vi "Lockin.DAQ.Read AI.vi"(8 "error in (no error)":errorcluster, 10 "AO []":waveform(dbl)[](array[waveform]), 11 "Lockin.DAQ in":refnum<class "Instrument.DAQ.lvclass">) -> (0 "error out":errorcluster, 1 "AI time (ms)":u32=2, 2 "AI []":waveform(dbl)[](array[waveform]), 3 "Lockin.DAQ out":refnum<class "Instrument.DAQ.lvclass">)   [LabVIEW 2019, in "Instrument.DAQ.lvclass"]
uses:
  Instrument.DAQ.lvclass
  Instrument.DAQ.lvclass/Instrument.DAQ.ctl
  Typedefs/AI Simulation-enum.ctl
  Waveguide Model/Waveguide Model--Cluster.ctl
  <vilib>/DAQmx/read.llb/DAQmx Read (Analog 1D Wfm NChan NSamp).vi
  <vilib>/DAQmx/miscellaneous.llb/DAQmx Fill In Error Info.vi
  <userlib>/_OpenG.lib/array/array.llb/Reorder 1D Array2 (Variant)__ogtk.vi
  <userlib>/_OpenG.lib/array/array.llb/Sort 1D Array (I32)__ogtk.vi
  <resource>/objmgr/daqmx.rc
panel:
  out "P Check":bool[](array[boolean])
  out "time to read samples":u32
  out "time to check for samples":u32
  out "Numeric":i32
  out "AvailSampPerChan 4":u32
  out "AvailSampPerChan 3":u32
  out "AvailSampPerChan 2":u32
  out "AvailSampPerChan 1":u32
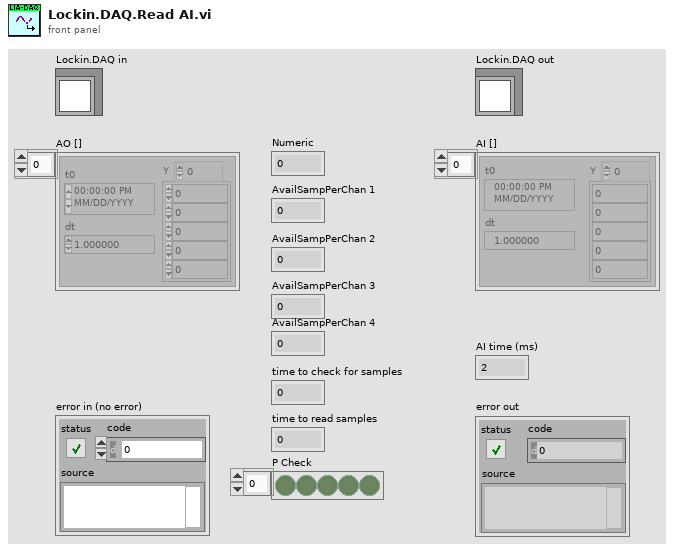
[diagram p1: front panel]
types:
  T1 = typedef "Instrument.DAQ.lvclass/AI Simulation-enum.ctl" = enum16{"AI = HW simulated", "AI = noise*AO", "AI = waveguide"}
  T2 = typedef "Instrument.DAQ.lvclass/Waveguide Model--Cluster.ctl" = cluster{"Vsource Index":i32, "Vsg Index":i32, "V+":i32, "V-":i32}
  T3 = enum16{"static", "dynamic", "dynamic asynchronous"}
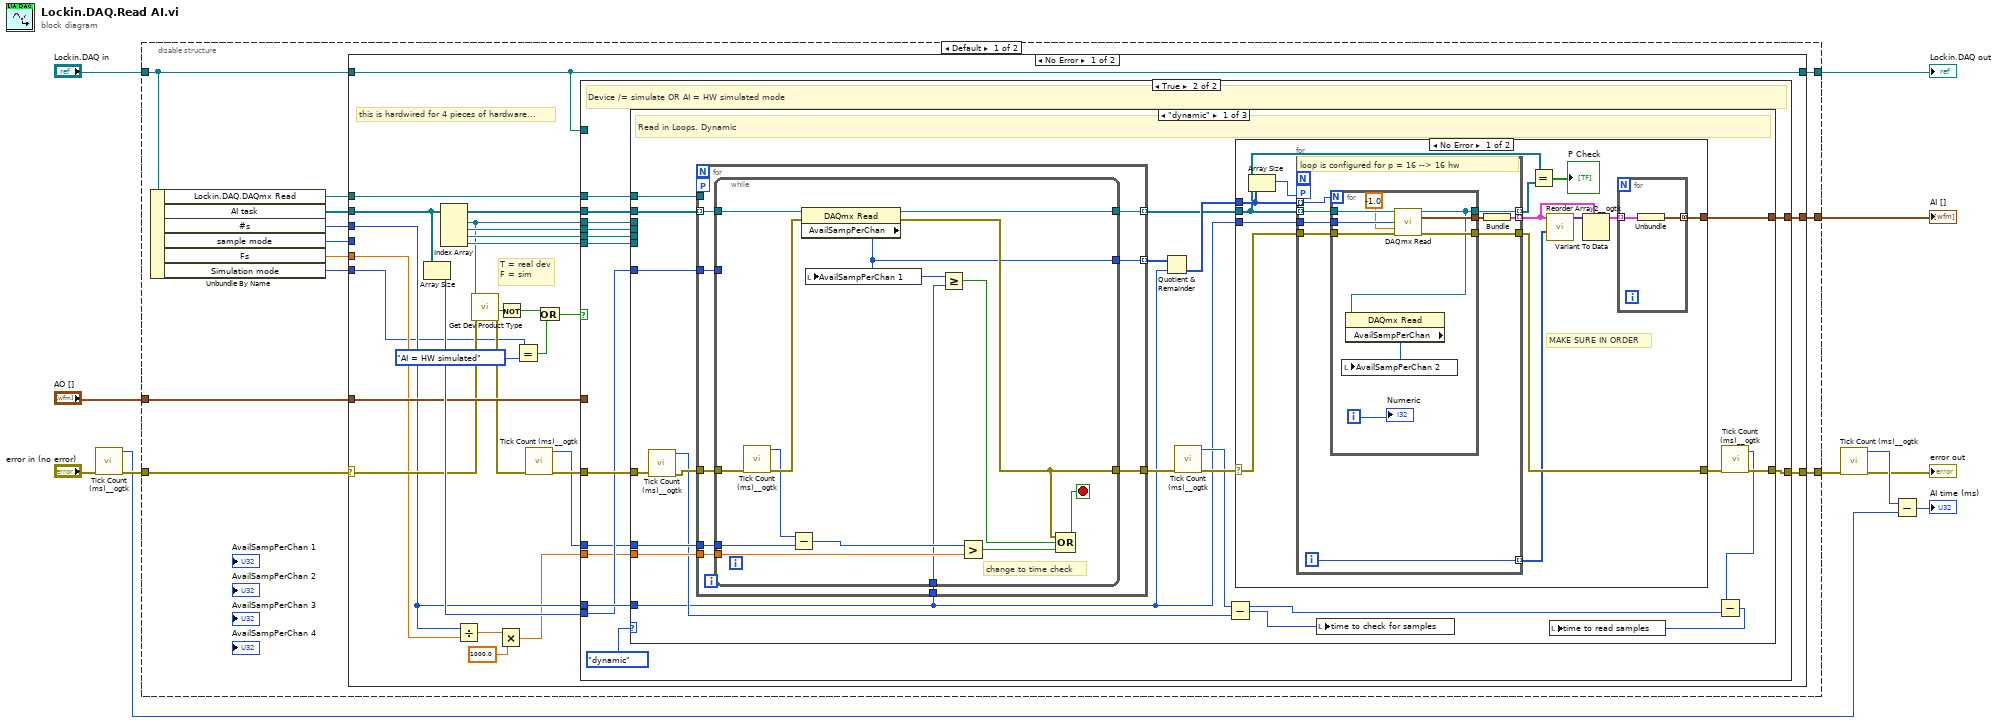
[diagram p0: block diagram]
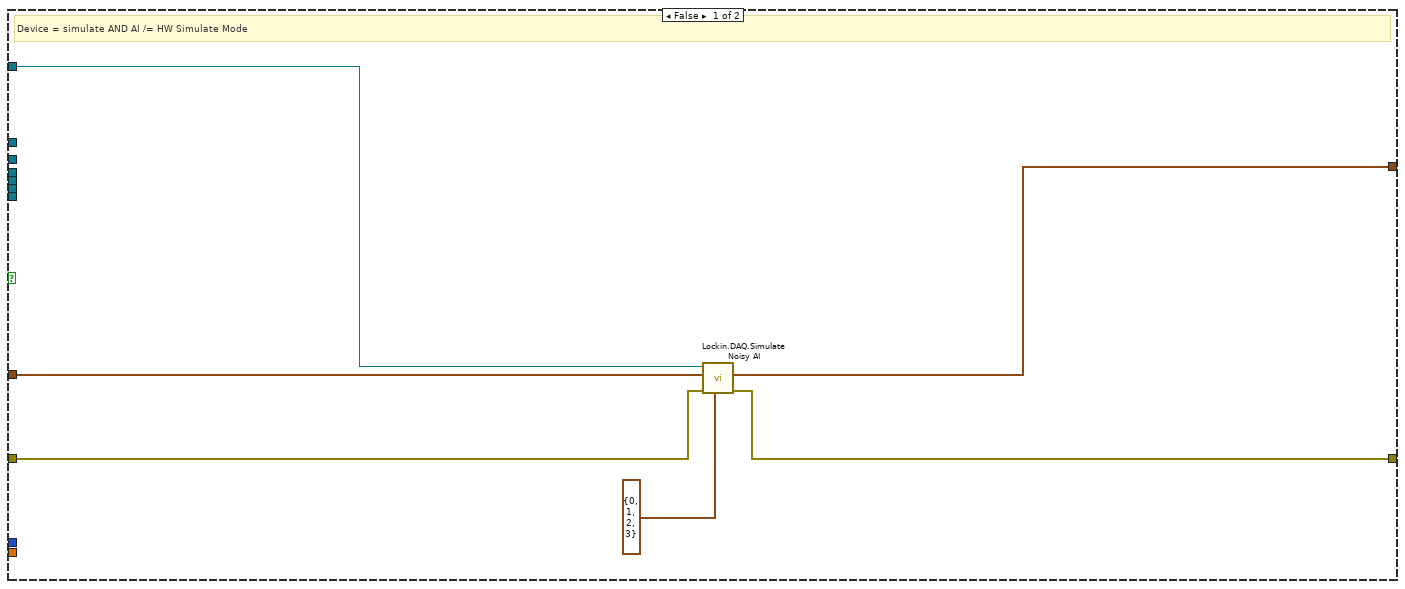
[diagram p2: hidden frame]
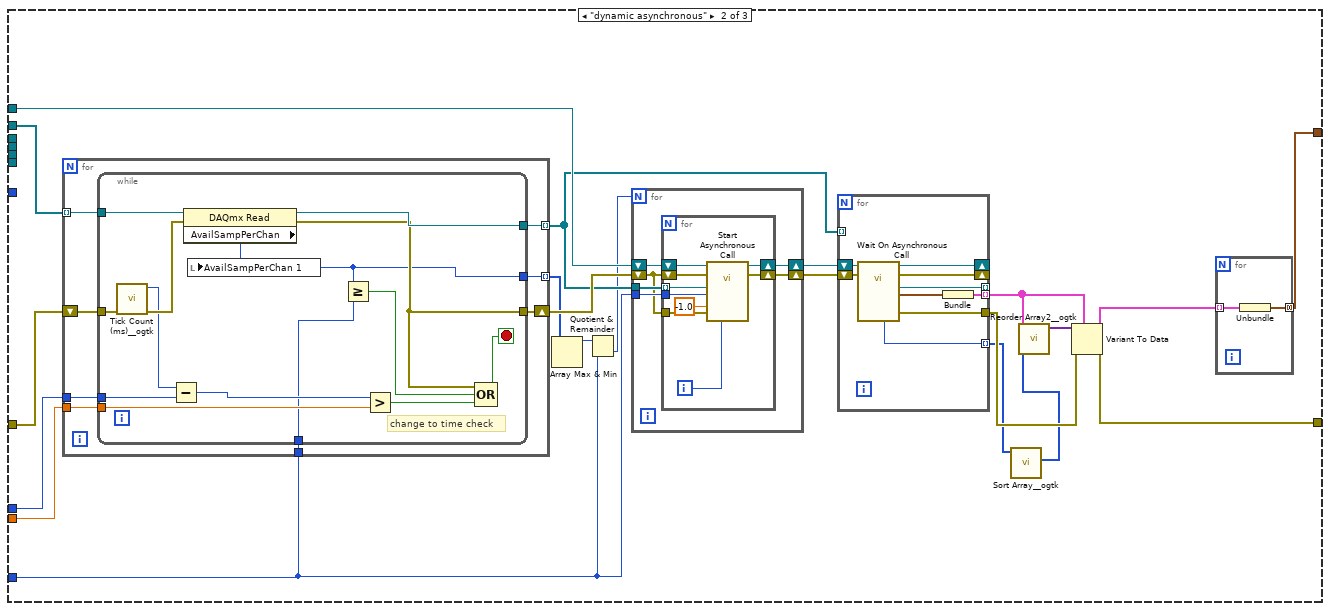
[diagram p4: hidden frame]
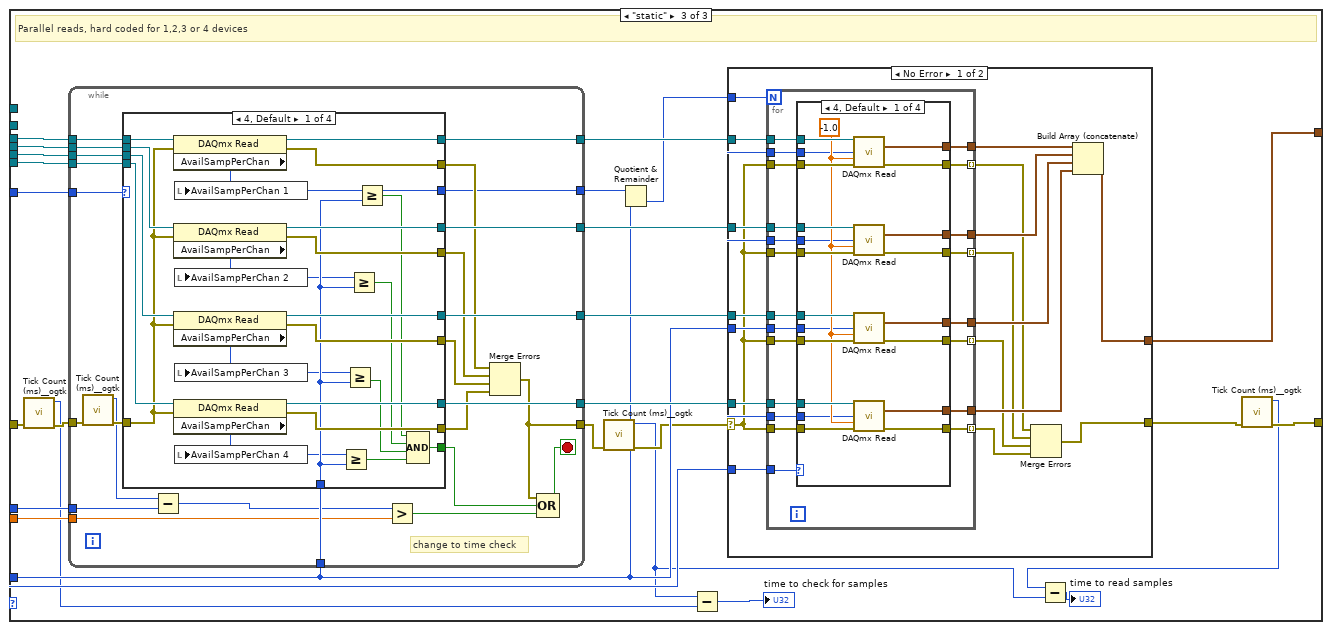
[diagram p5: hidden frame]
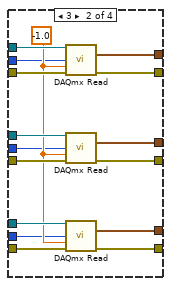
[diagram p6: hidden frame]
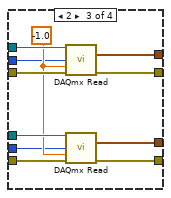
[diagram p7: hidden frame]
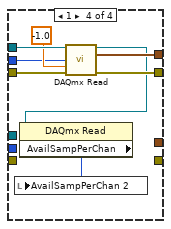
[diagram p8: hidden frame]
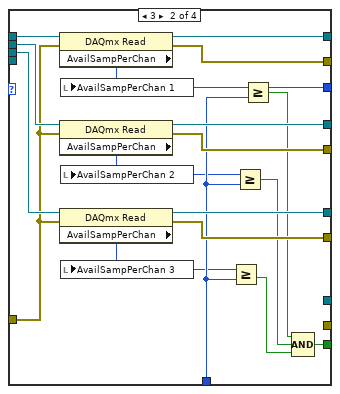
[diagram p10: hidden frame]
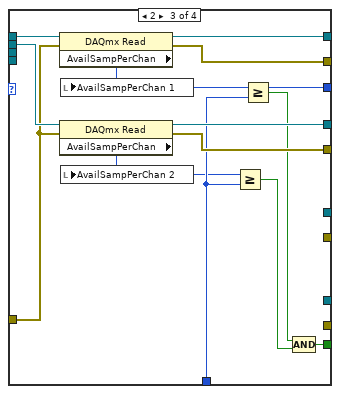
[diagram p11: hidden frame]
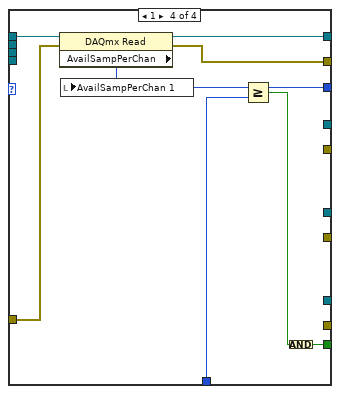
[diagram p12: hidden frame]
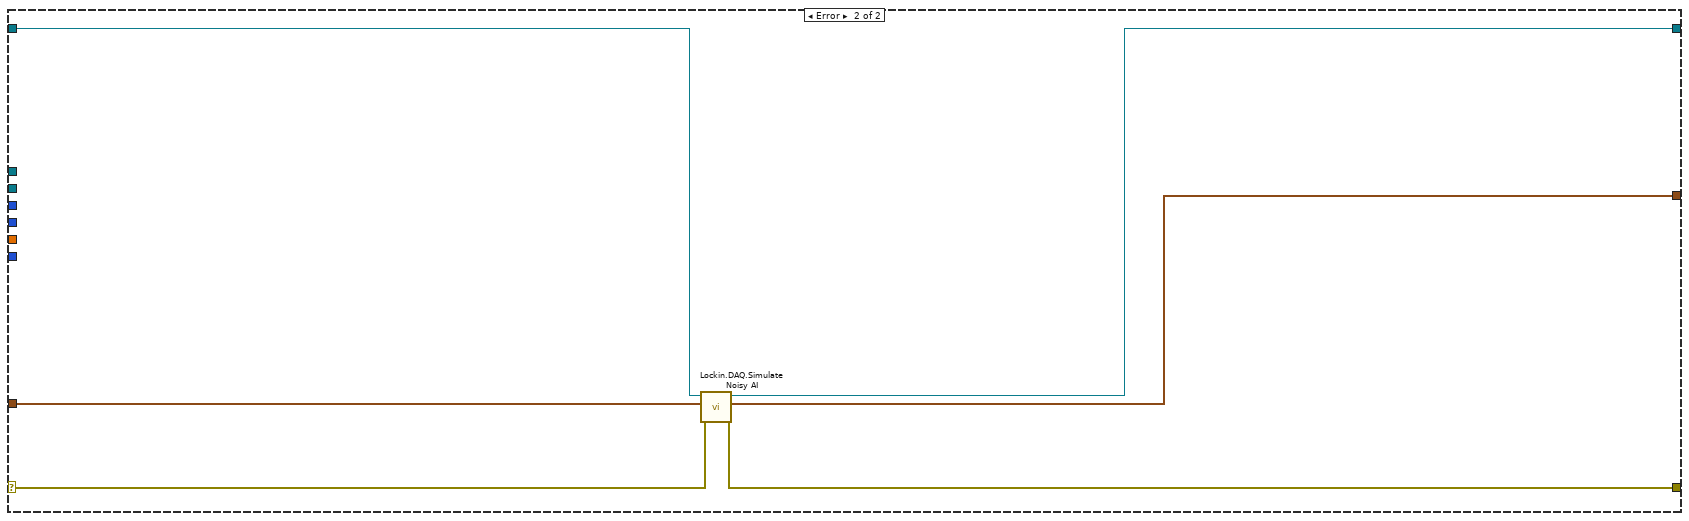
[diagram p13: hidden frame]
diagram:
  n1 = call <userlib>:"Tick Count (ms)__ogtk.vi"("error in (no error)"="error in (no error)") -> ("error out"=w8:errorcluster, "millisecond timer value"=w3:u32)  [unwired: 9 in]
  n2 = disable-structure shown="Default" {
    disable-tunnel: [w23 w432] -> w1
    disable-tunnel: [w20 w433] -> w7
    disable-tunnel: "Lockin.DAQ in" -> [w18 _]
    disable-tunnel: "AO []" -> [w19 w432]
    disable-tunnel: w8 -> [w14 w433]
    disable-tunnel: [w17 _] -> w10
    frame condition #0 (active) {
      n3 = Unbundle By Name(w18) -> ("Lockin.DAQ.DAQmx Read"=w13:refnum<vi>, "AI task"=w16:refnum<k21>[], "#s"=w22:i32, "sample mode"=w21:i32, "Fs"=w15:dbl, "Simulation mode"=w12:T1)
      n4 = case shown="No Error" w14 {
        selector: w14 -> [w40 w427]
        tunnel: [w49 w430] -> w23
        tunnel: w22 -> [w39 _]
        tunnel: w21 -> [_ _]
        tunnel: [w41 w429] -> w20
        tunnel: w19 -> [w44 w428]
        tunnel: w16 -> [w31 _]
        tunnel: w18 -> [w43 w426]
        tunnel: [w43 w431] -> w17
        tunnel: w15 -> [w38 _]
        tunnel: w13 -> [w30 _]
        tunnel: w12 -> [w24 _]
        frame No Error {
          # "T = real dev\nF = sim"
          # "this is hardwired for 4 pieces of hardware..."
          n5 = Array Size(array=w31) -> (size(s)=w45:i32)
          n6 = Index Array(array=w31) -> (element #1=w42:refnum<k21>, element #2=w46:refnum<k21>, element #3=w47:refnum<k21>, element #4=w48:refnum<k21>)  [unwired: 4 in]
          n7 = Divide(x=w39, y=w38) -> (x/y=w37:dbl)
          n8 = call "Get Dev Product Type.vi"("error in (no error)"=w40, "Refnum in"=w42) -> ("error out"=w34:errorcluster, "DevIsSimulated"=w27:bool)  [unwired: 6 in, 2 out]
          n9 = Multiply(x=w37, y=1000.0) -> (x*y=w33:dbl)
          n10 = Not(x=w27) -> (.not. x?=w25:bool)
          n11 = Equal?(x=w24, y=AI_Simulation-enum."AI = HW simulated") -> (x = y?=w28:bool)
          n12 = call <userlib>:"Tick Count (ms)__ogtk.vi"("error in (no error)"=w34) -> ("error out"=w35:errorcluster, "millisecond timer value"=w32:u32)  [unwired: 9 in]
          n13 = Or(x=w25, y=w28) -> (x .or. y?=w26:bool)
          n14 = case shown="True" w26 {
            tunnel: [w53 w69] -> w49
            tunnel: w48 -> [_ w68]
            tunnel: w47 -> [_ w67]
            tunnel: w46 -> [_ w66]
            tunnel: w42 -> [_ w65]
            tunnel: w39 -> [_ w64]
            tunnel: w35 -> [w51 w62]
            tunnel: w45 -> [_ w61]
            tunnel: [w50 w63] -> w41
            tunnel: w44 -> [w55 _]
            tunnel: w43 -> [w54 _]
            tunnel: w33 -> [_ w60]
            tunnel: w32 -> [_ w59]
            tunnel: w31 -> [_ w58]
            tunnel: w30 -> [_ w57]
            frame False {
              # "Device = simulate AND AI /= HW Simulate Mode"
              n15 = call "Lockin.DAQ.Simulate Noisy AI.vi"("Waveguide Cluster"=T2 {"Vsource Index"=0, "Vsg Index"=1, "V+"=2, "V-"=3}, "error in (no error)"=w51, "AO []"=w55, "Lockin.DAQ in"=w54) -> ("error out"=w50:errorcluster, "Noisy AI []"=w53:waveform(dbl)[])  [unwired: 5 in, 1 out]
            }
            frame True {
              # "Device /= simulate OR AI = HW simulated mode"
              n16 = case shown="\"dynamic\"" T3."dynamic" ("Enum") {
                tunnel: [w90 w166 w242] -> w69
                tunnel: w68 -> [_ _ w241]
                tunnel: w67 -> [_ _ w240]
                tunnel: w66 -> [_ _ w239]
                tunnel: w65 -> [_ _ w238]
                tunnel: w64 -> [w70 w157 w233]
                tunnel: [w79 w150 w221] -> w63
                tunnel: w62 -> [w81 w163 w225]
                tunnel: w61 -> [w85 _ w232]
                tunnel: w60 -> [w89 w161 w231]
                tunnel: w59 -> [w86 w162 w228]
                tunnel: w58 -> [w84 w165 _]
                tunnel: w57 -> [w82 w160 _]
                frame "dynamic" {
                  # "Read in Loops. Dynamic"
                  n17 = call <userlib>:"Tick Count (ms)__ogtk.vi"("error in (no error)"=w81) -> ("error out"=w80:errorcluster, "millisecond timer value"=w75:u32)  [unwired: 9 in]
                  n18 = for {
                    tunnel: w70 -> [w99]
                    tunnel: w89 -> [w97]
                    tunnel: w85 -> [w93]
                    tunnel: w84 -> [w92] mode=indexing
                    tunnel: w86 -> [w94]
                    tunnel: [w96] -> w87 mode=indexing
                    tunnel: [w91] -> w83 mode=indexing
                    tunnel: w82 -> [_]
                    workers-P: _ -> [_]
                    tunnel: w80 -> [w98]
                    tunnel: [w95] -> w78
                    n19 = while {
                      tunnel: [w113] -> w91
                      tunnel: w98 -> [w108]
                      tunnel: [w111] -> w95
                      tunnel: w99 -> [w100]
                      tunnel: w93 -> [_]
                      tunnel: w97 -> [w109]
                      tunnel: [w101] -> w96
                      tunnel: w94 -> [w105]
                      tunnel: w92 -> [w102]
                      stop <- w112 stop-if-true
                      # "change to time check"
                      n20 = call <userlib>:"Tick Count (ms)__ogtk.vi"("error in (no error)"=w108) -> ("error out"=w107:errorcluster, "millisecond timer value"=w106:u32)  [unwired: 9 in]
                      n21 = Subtract(x=w106, y=w105) -> (x-y=w104:u32)
                      n22 = property class="DAQmx Read"(reference=w102, error in=w107) -> (reference out=w113:refnum<k21>, error out=w111:errorcluster, "AvailSampPerChan"=w101:u32)
                      n23 = local write "AvailSampPerChan 1"(w101) -> ()
                      n24 = Greater Or Equal?(x=w101, y=w100) -> (x >= y?=w103:bool)
                      n25 = Greater?(x=w104, y=w109) -> (0:w110:bool)
                      n26 = Compound Arithmetic op=OR(w111, w103, w110) -> (w112:bool)
                    }
                  }
                  n27 = Quotient & Remainder(x=w87, y=w70) -> (floor(x/y)=w88:u32[])  [unwired: 1 out]
                  n28 = call <userlib>:"Tick Count (ms)__ogtk.vi"("error in (no error)"=w78) -> ("error out"=w77:errorcluster, "millisecond timer value"=w71:u32)  [unwired: 9 in]
                  n29 = Subtract(x=w71, y=w75) -> (x-y=w73:u32)
                  n30 = case shown="No Error" w77 {
                    selector: w77 -> [w125 w147]
                    tunnel: [w118 _] -> w90
                    tunnel: w70 -> [w126 _]
                    tunnel: [w122 w147] -> w76
                    tunnel: w88 -> [w124 _]
                    tunnel: w83 -> [w115 _]
                    frame No Error {
                      # "MAKE SURE IN ORDER"
                      n31 = Array Size(array=w124) -> (size(s)=w123:i32)
                      n32 = for {
                        N: w123 -> [_]
                        tunnel: w126 -> [w137]
                        tunnel: [w130] -> w117 mode=indexing
                        tunnel: w124 -> [w132] mode=indexing
                        tunnel: w125 -> [w135]
                        tunnel: [w134] -> w122
                        tunnel: w115 -> [w133] mode=indexing
                        workers-P: w123 -> [_]
                        tunnel: [w131] -> w119 mode=indexing
                        tunnel: [w129] -> w116 mode=indexing
                        i -> [w131]
                        # "loop is configured for p = 16 --> 16 hw"
                        n33 = for {
                          N: w132 -> [_]
                          tunnel: w133 -> [w146]
                          tunnel: w135 -> [w145]
                          tunnel: [w144] -> w136
                          tunnel: w137 -> [w143]
                          tunnel: [w142] -> w134
                          tunnel: [w138] -> w129
                          i -> [w141]
                          n34 = call-poly <vilib>:"DAQmx Read.vi"("task/channels in"=w146, "number of samples per channel"=w143, "timeout"=-1.0, "error in"=w145) -> ("task out"=w138:refnum<k21>, "data"=w144:waveform(dbl)[], "error out"=w142:errorcluster)  [unwired: 9 in]
                          n35 = property class="DAQmx Read"(reference=w138) -> ("AvailSampPerChan"=w139:u32)  [unwired: 1 in, 2 out]
                          n36 = local write "AvailSampPerChan 2"(w139) -> ()
                          "Numeric" <- w141
                        }
                        n37 = Bundle("data"=w136) -> (w130:cluster{"data":waveform(dbl)[]})  [unwired: 1 in]
                      }
                      n38 = Equal?(x=w115, y=w116) -> (x = y?=→"P Check":bool[])
                      n39 = call-poly <userlib>:"Reorder Array2__ogtk.vi"("indices"=w119, "array"=w117) -> ("reordered array"=w121:variant[])  [unwired: 9 in]
                      n40 = Variant To Data(type=w117, Variant=w121) -> (data=w120:cluster{"data":waveform(dbl)[]}[])  [unwired: 1 in, 1 out]
                      n41 = for {
                        tunnel: w120 -> [w128] mode=indexing
                        tunnel: [w127] -> w118 mode=concatenating
                        n42 = Unbundle(w128) -> ("data"=w127:waveform(dbl)[])
                      }
                    }
                    frame Error {
                    }
                  }
                  n43 = local write "time to check for samples"(w73) -> ()
                  n44 = call <userlib>:"Tick Count (ms)__ogtk.vi"("error in (no error)"=w76) -> ("error out"=w79:errorcluster, "millisecond timer value"=w74:u32)  [unwired: 9 in]
                  n45 = Subtract(x=w74, y=w71) -> (x-y=w72:u32)
                  n46 = local write "time to read samples"(w72) -> ()
                }
                frame "dynamic asynchronous" {
                  n47 = for {
                    tunnel: w157 -> [w191]
                    tunnel: w161 -> [w189]
                    shift-right: [w187] -> w164
                    shift-left: w163 -> [w190]
                    tunnel: w165 -> [w185] mode=indexing
                    tunnel: w162 -> [w186]
                    tunnel: [w188] -> w159 mode=indexing
                    tunnel: [w184] -> w156 mode=indexing
                    n48 = while {
                      tunnel: [w205] -> w184
                      tunnel: w190 -> [w200]
                      tunnel: [w203] -> w187
                      tunnel: w191 -> [w192]
                      tunnel: w189 -> [w201]
                      tunnel: [w193] -> w188
                      tunnel: w186 -> [w197]
                      tunnel: w185 -> [w194]
                      stop <- w204 stop-if-true
                      # "change to time check"
                      n49 = call <userlib>:"Tick Count (ms)__ogtk.vi"("error in (no error)"=w200) -> ("error out"=w199:errorcluster, "millisecond timer value"=w198:u32)  [unwired: 9 in]
                      n50 = Subtract(x=w198, y=w197) -> (x-y=w196:u32)
                      n51 = property class="DAQmx Read"(reference=w194, error in=w199) -> (reference out=w205:refnum<k21>, error out=w203:errorcluster, "AvailSampPerChan"=w193:u32)
                      n52 = local write "AvailSampPerChan 1"(w193) -> ()
                      n53 = Greater Or Equal?(x=w193, y=w192) -> (x >= y?=w195:bool)
                      n54 = Greater?(x=w196, y=w201) -> (0:w202:bool)
                      n55 = Compound Arithmetic op=OR(w203, w195, w202) -> (w204:bool)
                    }
                  }
                  n56 = Array Max & Min(array=w159) -> (max value=w158:u32)  [unwired: 3 out]
                  n57 = Quotient & Remainder(x=w158, y=w157) -> (floor(x/y)=w155:u32)  [unwired: 1 out]
                  n58 = for {
                    N: w155 -> [_]
                    tunnel: w156 -> [w172]
                    tunnel: w157 -> [w170]
                    shift-right: [w173] -> w167
                    shift-left: w164 -> [w169]
                    shift-right: [w174] -> w168
                    shift-left: w160 -> [w171]
                    n59 = for {
                      shift-right: [w183] -> w173
                      shift-left: w169 -> [w180]
                      shift-right: [w182] -> w174
                      shift-left: w171 -> [w181]
                      tunnel: w169 -> [w179]
                      tunnel: w172 -> [w178] mode=indexing
                      tunnel: w170 -> [w176]
                      i -> [w175]
                      n60 = call-by-ref "Start Asynchronous Call"(reference=w181, error in=w180, "Refnum in"=w178, "number of samples per channel"=w176, "timeout"=-1.0, 11:"error in (no error)"=w179, "ID in"=w175) -> (reference out=w182:refnum<vi>, error out=w183:errorcluster)  [unwired: 7 in, 4 out]
                    }
                  }
                  n61 = for {
                    shift-right: [w211] -> _
                    shift-left: w167 -> [w213]
                    shift-right: [w212] -> _
                    shift-left: w168 -> [w214]
                    tunnel: [w208] -> _ mode=indexing
                    tunnel: [w210] -> w151
                    tunnel: [w207] -> w153 mode=indexing
                    tunnel: [w206] -> w149 mode=indexing
                    tunnel: w156 -> [_] mode=indexing
                    n62 = call-by-ref "Wait On Asynchronous Call"(reference=w214, error in=w213) -> (reference out=w212:refnum<vi>, error out=w211:errorcluster, "Refnum out"=w208:refnum<k21>, "data"=w209:waveform(dbl)[], "ID out"=w206:i32, 15:"error out"=w210:errorcluster)  [unwired: 12 in]
                    n63 = Bundle("data"=w209) -> (w207:cluster{"data":waveform(dbl)[]})  [unwired: 1 in]
                  }
                  n64 = call-poly <userlib>:"Sort Array__ogtk.vi"("Array in"=w149) -> ("Sorted Pointers"=w148:i32[])  [unwired: 9 in, 1 out]
                  n65 = call-poly <userlib>:"Reorder Array2__ogtk.vi"("indices"=w148, "array"=w153) -> ("reordered array"=w154:variant[])  [unwired: 9 in]
                  n66 = Variant To Data(error in=w151, type=w153, Variant=w154) -> (data=w152:cluster{"data":waveform(dbl)[]}[], error out=w150:errorcluster)
                  n67 = for {
                    tunnel: [w216] -> w166 mode=concatenating
                    tunnel: w152 -> [w215] mode=indexing
                    n68 = Unbundle(w215) -> ("data"=w216:waveform(dbl)[])
                  }
                }
                frame "static" {
                  # "Parallel reads, hard coded for 1,2,3 or 4 devices"
                  n69 = call <userlib>:"Tick Count (ms)__ogtk.vi"("error in (no error)"=w225) -> ("error out"=w224:errorcluster, "millisecond timer value"=w223:u32)  [unwired: 9 in]
                  n70 = while {
                    tunnel: w241 -> [w363]
                    tunnel: w240 -> [w362]
                    tunnel: w239 -> [w361]
                    tunnel: w238 -> [w360]
                    tunnel: [w359] -> w237
                    tunnel: [w358] -> w236
                    tunnel: [w357] -> w235
                    tunnel: [w356] -> w234
                    tunnel: w224 -> [w343]
                    tunnel: [w345] -> w227
                    tunnel: w233 -> [w355]
                    tunnel: w232 -> [w354]
                    tunnel: w231 -> [w347]
                    tunnel: [w344] -> w229
                    tunnel: w228 -> [w340]
                    stop <- w353 stop-if-true
                    # "change to time check"
                    n71 = call <userlib>:"Tick Count (ms)__ogtk.vi"("error in (no error)"=w343) -> ("error out"=w342:errorcluster, "millisecond timer value"=w341:u32)  [unwired: 9 in]
                    n72 = case shown="4, Default" w354 {
                      tunnel: w363 -> [w386 _ _ _]
                      tunnel: w362 -> [w385 w404 _ _]
                      tunnel: w361 -> [w384 w403 w417 _]
                      tunnel: w360 -> [w383 w402 w416 w425]
                      tunnel: [w382 w401 w415 w424] -> w359
                      tunnel: [w381 w400 w414 _] -> w358
                      tunnel: [w380 w399 _ _] -> w357
                      tunnel: [w379 _ _ _] -> w356
                      tunnel: [w378 w398 w413 w423] -> w349
                      tunnel: [w377 w397 w412 _] -> w350
                      tunnel: [w376 w396 _ _] -> w351
                      tunnel: [w375 _ _ _] -> w352
                      tunnel: w342 -> [w374 w395 w411 w422]
                      tunnel: w355 -> [w369 w391 w408 w420]
                      tunnel: [w365 w388 w406 w419] -> w346
                      tunnel: [w364 w387 w405 w418] -> w344
                      frame 4, Default {
                        n73 = property class="DAQmx Read"(reference=w383, error in=w374) -> (reference out=w382:refnum<k21>, error out=w378:errorcluster, "AvailSampPerChan"=w364:u32)
                        n74 = property class="DAQmx Read"(reference=w384, error in=w374) -> (reference out=w381:refnum<k21>, error out=w377:errorcluster, "AvailSampPerChan"=w366:u32)
                        n75 = property class="DAQmx Read"(reference=w385, error in=w374) -> (reference out=w380:refnum<k21>, error out=w376:errorcluster, "AvailSampPerChan"=w367:u32)
                        n76 = property class="DAQmx Read"(reference=w386, error in=w374) -> (reference out=w379:refnum<k21>, error out=w375:errorcluster, "AvailSampPerChan"=w368:u32)
                        n77 = local write "AvailSampPerChan 1"(w364) -> ()
                        n78 = local write "AvailSampPerChan 2"(w366) -> ()
                        n79 = local write "AvailSampPerChan 3"(w367) -> ()
                        n80 = local write "AvailSampPerChan 4"(w368) -> ()
                        n81 = Greater Or Equal?(x=w368, y=w369) -> (x >= y?=w373:bool)
                        n82 = Greater Or Equal?(x=w367, y=w369) -> (x >= y?=w372:bool)
                        n83 = Greater Or Equal?(x=w366, y=w369) -> (x >= y?=w371:bool)
                        n84 = Greater Or Equal?(x=w364, y=w369) -> (x >= y?=w370:bool)
                        n85 = Compound Arithmetic op=AND(w370, w371, w372, w373) -> (w365:bool)
                      }
                      frame 3 {
                        n86 = property class="DAQmx Read"(reference=w402, error in=w395) -> (reference out=w401:refnum<k21>, error out=w398:errorcluster, "AvailSampPerChan"=w387:u32)
                        n87 = property class="DAQmx Read"(reference=w403, error in=w395) -> (reference out=w400:refnum<k21>, error out=w397:errorcluster, "AvailSampPerChan"=w389:u32)
                        n88 = property class="DAQmx Read"(reference=w404, error in=w395) -> (reference out=w399:refnum<k21>, error out=w396:errorcluster, "AvailSampPerChan"=w390:u32)
                        n89 = local write "AvailSampPerChan 1"(w387) -> ()
                        n90 = local write "AvailSampPerChan 2"(w389) -> ()
                        n91 = local write "AvailSampPerChan 3"(w390) -> ()
                        n92 = Greater Or Equal?(x=w390, y=w391) -> (x >= y?=w394:bool)
                        n93 = Greater Or Equal?(x=w389, y=w391) -> (x >= y?=w393:bool)
                        n94 = Greater Or Equal?(x=w387, y=w391) -> (x >= y?=w392:bool)
                        n95 = Compound Arithmetic op=AND(w392, w393, w394) -> (w388:bool)
                      }
                      frame 2 {
                        n96 = property class="DAQmx Read"(reference=w416, error in=w411) -> (reference out=w415:refnum<k21>, error out=w413:errorcluster, "AvailSampPerChan"=w405:u32)
                        n97 = property class="DAQmx Read"(reference=w417, error in=w411) -> (reference out=w414:refnum<k21>, error out=w412:errorcluster, "AvailSampPerChan"=w407:u32)
                        n98 = local write "AvailSampPerChan 1"(w405) -> ()
                        n99 = local write "AvailSampPerChan 2"(w407) -> ()
                        n100 = Greater Or Equal?(x=w407, y=w408) -> (x >= y?=w410:bool)
                        n101 = Greater Or Equal?(x=w405, y=w408) -> (x >= y?=w409:bool)
                        n102 = Compound Arithmetic op=AND(w409, w410) -> (w406:bool)
                      }
                      frame 1 {
                        n103 = property class="DAQmx Read"(reference=w425, error in=w422) -> (reference out=w424:refnum<k21>, error out=w423:errorcluster, "AvailSampPerChan"=w418:u32)
                        n104 = local write "AvailSampPerChan 1"(w418) -> ()
                        n105 = Greater Or Equal?(x=w418, y=w420) -> (x >= y?=w421:bool)
                        n106 = Compound Arithmetic op=AND(w421) -> (w419:bool)
                      }
                    }
                    n107 = Subtract(x=w341, y=w340) -> (x-y=w339:u32)
                    n108 = Greater?(x=w339, y=w347) -> (0:w348:bool)
                    n109 = Merge Errors(w349, w350, w351, w352) -> (w345:errorcluster)
                    n110 = Compound Arithmetic op=OR(w345, w346, w348) -> (w353:bool)
                  }
                  n111 = call <userlib>:"Tick Count (ms)__ogtk.vi"("error in (no error)"=w227) -> ("error out"=w226:errorcluster, "millisecond timer value"=w218:u32)  [unwired: 9 in]
                  n112 = Quotient & Remainder(x=w229, y=w233) -> (floor(x/y)=w230:u32)  [unwired: 1 out]
                  n113 = Subtract(x=w218, y=w223) -> (x-y=→"time to check for samples":u32)
                  n114 = case shown="No Error" w226 {
                    selector: w226 -> [w243 w338]
                    tunnel: [w260 _] -> w242
                    tunnel: w237 -> [w259 _]
                    tunnel: w236 -> [w258 _]
                    tunnel: w235 -> [w257 _]
                    tunnel: w234 -> [w256 _]
                    tunnel: w233 -> [w252 _]
                    tunnel: [w247 w338] -> w222
                    tunnel: w232 -> [w245 _]
                    tunnel: w230 -> [w244 _]
                    frame No Error {
                      n115 = for {
                        N: w244 -> [_]
                        tunnel: w259 -> [w281]
                        tunnel: w258 -> [w280]
                        tunnel: w257 -> [w279]
                        tunnel: w256 -> [w278]
                        tunnel: w243 -> [w277]
                        tunnel: w243 -> [w276]
                        tunnel: w243 -> [w275]
                        tunnel: w243 -> [w274]
                        tunnel: [w273] -> w255
                        tunnel: [w272] -> w246
                        tunnel: [w271] -> w254
                        tunnel: [w270] -> w253
                        tunnel: w252 -> [w269]
                        tunnel: w252 -> [w268]
                        tunnel: w252 -> [w267]
                        tunnel: w252 -> [w266]
                        tunnel: [w265] -> w251 mode=indexing
                        tunnel: [w264] -> w250 mode=indexing
                        tunnel: [w263] -> w249 mode=indexing
                        tunnel: [w262] -> w248 mode=indexing
                        tunnel: w245 -> [w261]
                        n116 = case shown="4, Default" w261 {
                          tunnel: w281 -> [w302 w318 w329 w337]
                          tunnel: w280 -> [w301 w317 w328 _]
                          tunnel: w279 -> [w300 w316 _ _]
                          tunnel: w278 -> [w299 _ _ _]
                          tunnel: w277 -> [w298 w315 w327 w336]
                          tunnel: w276 -> [w297 w314 w326 _]
                          tunnel: w275 -> [w296 w313 _ _]
                          tunnel: w274 -> [w295 _ _ _]
                          tunnel: [w293 w311 w324 _] -> w273
                          tunnel: [w292 w310 w323 w334] -> w272
                          tunnel: [w291 w309 _ _] -> w271
                          tunnel: [w290 _ _ _] -> w270
                          tunnel: w269 -> [w289 _ _ _]
                          tunnel: w268 -> [w288 w308 w322 w333]
                          tunnel: w267 -> [w287 w307 _ _]
                          tunnel: w266 -> [w286 w306 w321 _]
                          tunnel: [w285 w305 w320 w332] -> w265
                          tunnel: [w284 w304 w319 _] -> w264
                          tunnel: [w283 w303 _ _] -> w263
                          tunnel: [w282 _ _ _] -> w262
                          frame 4, Default {
                            w294 = -1.0 ("timeout")
                            n117 = call-poly <vilib>:"DAQmx Read.vi"("task/channels in"=w302, "number of samples per channel"=w288, "timeout"=w294, "error in"=w298) -> ("data"=w292:waveform(dbl)[], "error out"=w285:errorcluster)  [unwired: 9 in, 1 out]
                            n118 = call-poly <vilib>:"DAQmx Read.vi"("task/channels in"=w301, "number of samples per channel"=w286, "timeout"=w294, "error in"=w297) -> ("data"=w293:waveform(dbl)[], "error out"=w284:errorcluster)  [unwired: 9 in, 1 out]
                            n119 = call-poly <vilib>:"DAQmx Read.vi"("task/channels in"=w300, "number of samples per channel"=w287, "timeout"=w294, "error in"=w296) -> ("data"=w291:waveform(dbl)[], "error out"=w283:errorcluster)  [unwired: 9 in, 1 out]
                            n120 = call-poly <vilib>:"DAQmx Read.vi"("task/channels in"=w299, "number of samples per channel"=w289, "timeout"=w294, "error in"=w295) -> ("data"=w290:waveform(dbl)[], "error out"=w282:errorcluster)  [unwired: 9 in, 1 out]
                          }
                          frame 3 {
                            w312 = -1.0 ("timeout")
                            n121 = call-poly <vilib>:"DAQmx Read.vi"("task/channels in"=w318, "number of samples per channel"=w308, "timeout"=w312, "error in"=w315) -> ("data"=w310:waveform(dbl)[], "error out"=w305:errorcluster)  [unwired: 9 in, 1 out]
                            n122 = call-poly <vilib>:"DAQmx Read.vi"("task/channels in"=w317, "number of samples per channel"=w306, "timeout"=w312, "error in"=w314) -> ("data"=w311:waveform(dbl)[], "error out"=w304:errorcluster)  [unwired: 9 in, 1 out]
                            n123 = call-poly <vilib>:"DAQmx Read.vi"("task/channels in"=w316, "number of samples per channel"=w307, "timeout"=w312, "error in"=w313) -> ("data"=w309:waveform(dbl)[], "error out"=w303:errorcluster)  [unwired: 9 in, 1 out]
                          }
                          frame 2 {
                            w325 = -1.0 ("timeout")
                            n124 = call-poly <vilib>:"DAQmx Read.vi"("task/channels in"=w329, "number of samples per channel"=w322, "timeout"=w325, "error in"=w327) -> ("data"=w323:waveform(dbl)[], "error out"=w320:errorcluster)  [unwired: 9 in, 1 out]
                            n125 = call-poly <vilib>:"DAQmx Read.vi"("task/channels in"=w328, "number of samples per channel"=w321, "timeout"=w325, "error in"=w326) -> ("data"=w324:waveform(dbl)[], "error out"=w319:errorcluster)  [unwired: 9 in, 1 out]
                          }
                          frame 1 {
                            n126 = call-poly <vilib>:"DAQmx Read.vi"("task/channels in"=w337, "number of samples per channel"=w333, "timeout"=-1.0, "error in"=w336) -> ("task out"=w330:refnum<k21>, "data"=w334:waveform(dbl)[], "error out"=w332:errorcluster)  [unwired: 9 in]
                            n127 = property class="DAQmx Read"(reference=w330) -> ("AvailSampPerChan"=w331:u32)  [unwired: 1 in, 2 out]
                            n128 = local write "AvailSampPerChan 2"(w331) -> ()
                          }
                        }
                      }
                      n129 = Merge Errors(w251, w250, w249, w248) -> (w247:errorcluster)
                      n130 = Build Array (concatenate)(w246, w255, w254, w253) -> (w260:waveform(dbl)[])
                    }
                    frame Error {
                    }
                  }
                  n131 = call <userlib>:"Tick Count (ms)__ogtk.vi"("error in (no error)"=w222) -> ("error out"=w221:errorcluster, "millisecond timer value"=w220:u32)  [unwired: 9 in]
                  n132 = Subtract(x=w220, y=w218) -> (x-y=→"time to read samples":u32)
                }
              }
            }
          }
        }
        frame Error {
          n133 = call "Lockin.DAQ.Simulate Noisy AI.vi"("error in (no error)"=w427, "AO []"=w428, "Lockin.DAQ in"=w426) -> ("error out"=w429:errorcluster, "Noisy AI []"=w430:waveform(dbl)[], "Lockin.DAQ out"=w431:refnum<class "Instrument.DAQ.lvclass">)  [unwired: 6 in]
        }
      }
    }
    frame condition #1 {
    }
  }
  "AI []" <- w1
  "Lockin.DAQ out" <- w10
  n134 = call <userlib>:"Tick Count (ms)__ogtk.vi"("error in (no error)"=w7) -> ("error out"=→"error out":errorcluster, "millisecond timer value"=w6:u32)  [unwired: 9 in]
  n135 = Subtract(x=w6, y=w3) -> (x-y=→"AI time (ms)":u32)
